vi "dio64StartGF.vi"(9 "dio64 start":bool=TRUE, 10 "Action":enum16{"Write", "Read"}(ring)) -> (1 "dio64 started?":bool)   [LabVIEW 2009, in "Hardware.lvlib" / "Channels.lvlib"]
doc: "Is a global functional that tells other vi's whether or not the dio64 card is running or has stopped.\nThis is so that ni cards with external triggering know that they can stop, otherwise they will continue to run."
uses:
  Channels.lvlib
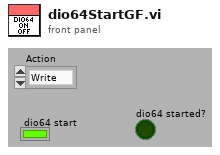
[diagram p1: front panel]
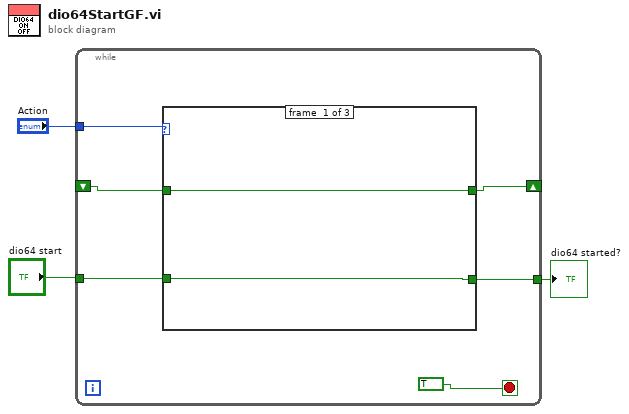
[diagram p0: block diagram]
diagram:
  n1 = while {
    tunnel: "Action" -> [w9]
    shift-right: [w5] -> _
    shift-left: _ -> [w7]
    tunnel: [w6] -> w1
    tunnel: "dio64 start" -> [w4]
    stop <- TRUE stop-if-true
    n2 = case shown="\"Write\"" w9 {
      tunnel: [w11 w12 w13] -> w5
      tunnel: w4 -> [w10 w12 _]
      tunnel: w7 -> [w11 _ w13]
      tunnel: [w10 w12 w13] -> w6
      frame #0 {
      }
      frame #1 {
      }
      frame #2 {
      }
    }
  }
  "dio64 started?" <- w1
